vi "Preview Store.vi"(6 "Local Data in":T1, 7 "Action":enum16{"Open", "Get", "Close"}(ring)=enum."Get", 8 "error in (no error)":errorcluster, 10 "% resolution":i32=10) -> (2 "Image Store":T8[][](array[typedef]), 4 "Local Data out":T1)   [LabVIEW 2024]
uses:
  Controls/Test Cluster.ctl
  Controls/Excluded Information.ctl
  Controls/Language.ctl
  Controls/Device_Type.ctl
  <vilib>/Utility/miscctls.llb/LVRectTypeDef.ctl
  <vilib>/Utility/miscctls.llb/LVBoundsTypeDef.ctl
  Controls/RVHR - Local Data.ctl
  <vilib>/picture/picture.llb/imagedata.ctl
panel:
  out "2D Picture":picture
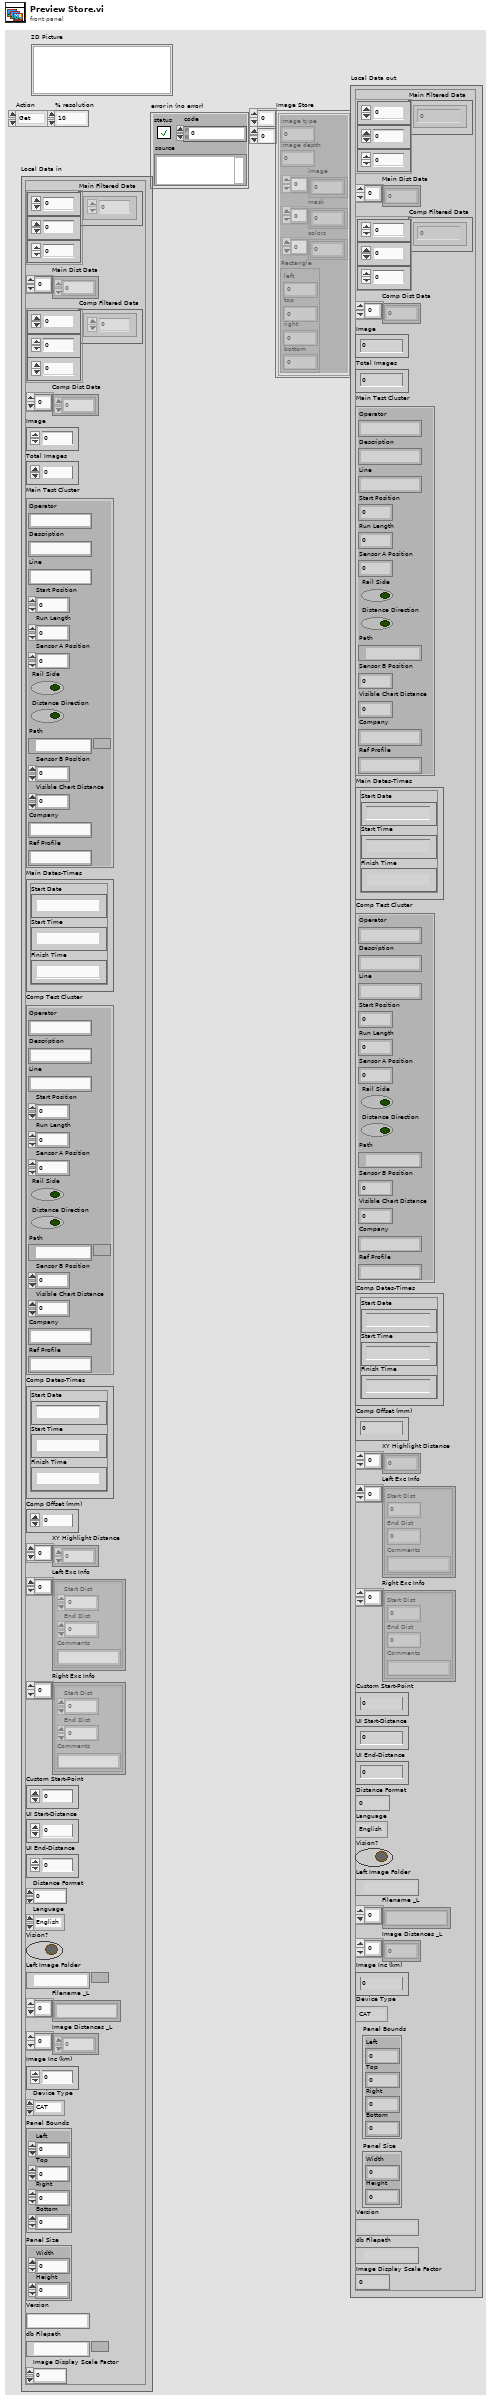
[diagram p1: front panel]
types:
  T1 = typedef "RVHR - Local Data.ctl" = cluster{"Main Filtered Data":dbl[][][], "Main Dist Data":dbl[], "Comp Filtered Data":dbl[][][], "Comp Dist Data":dbl[], "Image":u16, "Total Images":u16, "Main Test Cluster":T2, "Main Dates-Times":cluster{"Start Date":string, "Start Time":string, "Finish Time":string}, "Comp Test Cluster":T2, "Comp Dates-Times":cluster{"Start Date":string, "Start Time":string, "Finish Time":string}, "Comp Offset (mm)":i64, "XY Highlight Distance":dbl[], "Left Exc Info":T3[], "Right Exc Info":T3[], "Custom Start-Point":dbl, "UI Start-Distance":dbl, "UI End-Distance":dbl, "Distance Format":u8, "Language":T4, "Vision?":bool, "Left Image Folder":path, "Filename _L":string[], "Image Distances _L":dbl[], "Image Inc (km)":dbl, "Device Type":T5, "Panel Bounds":T6, "Panel Size":T7, "Version":string, "db Filepath":path, "Image Display Scale Factor":dbl}
  T2 = typedef "Test Cluster.ctl" = cluster{"Operator":string, "Description":string, "Line":string, "Start Position":dbl, "Run Length":dbl, "Sensor A Position":dbl, "Rail Side":bool, "Distance Direction":bool, "Path":path, "Sensor B Position":dbl, "Visible Chart Distance":dbl, "Company":string, "Ref Profile":string}
  T3 = typedef "Excluded Information.ctl" = cluster{"Start Dist":dbl, "End Dist":dbl, "Comments":string}
  T4 = typedef "Language.ctl" = enum16{"English", "Chinese", "German"}
  T5 = typedef "Device_Type.ctl" = enum16{"CAT", "Bi-CAT", "YRCA", "RCA", "RV-HR", "TV-HR"}
  T6 = typedef "LVRectTypeDef.ctl" = cluster{"Left":i16, "Top":i16, "Right":i16, "Bottom":i16}
  T7 = typedef "LVBoundsTypeDef.ctl" = cluster{"Width":u32, "Height":u32}
  T8 = typedef "imagedata.ctl" = cluster{"image type":i32, "image depth":i32, "image":u8[], "mask":u8[], "colors":u32[], "Rectangle":cluster{"left":i16, "top":i16, "right":i16, "bottom":i16}}
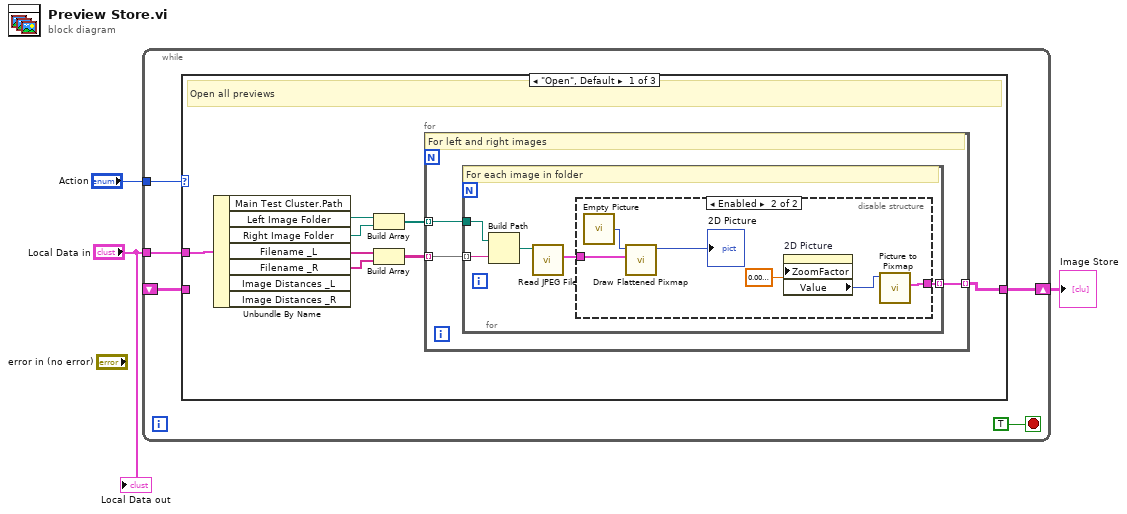
[diagram p0: block diagram]
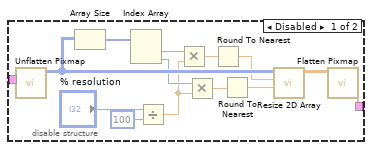
[diagram p2: hidden frame]
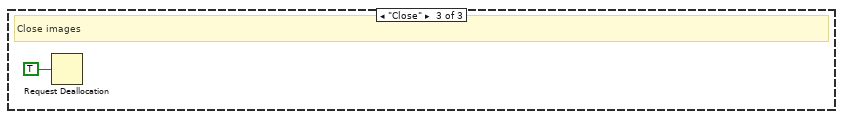
[diagram p4: hidden frame]
diagram:
  n1 = while {
    tunnel: "Action" -> [w8]
    tunnel: "Local Data in" -> [w7]
    shift-right: [w5] -> w1
    shift-left: _ -> [w4]
    stop <- TRUE stop-if-true
    n2 = case shown="\"Open\", Default" w8 {
      tunnel: w7 -> [w16 _ _]
      tunnel: [w9 w45 _] -> w5
      tunnel: w4 -> [_ w45 _]
      frame "Open", Default {
        # "Open all previews"
        n3 = Unbundle By Name(w16) -> ("Left Image Folder"=w12:path, "Right Image Folder"=w11:path, "Filename _L"=w15:string[], "Filename _R"=w14:string[])  [unwired: 3 out]
        n4 = Build Array(w12, w11) -> (w10:path[])
        n5 = Build Array(w15, w14) -> (w13:string[][])
        n6 = for {
          tunnel: w13 -> [w19] mode=indexing
          tunnel: w10 -> [w18] mode=indexing
          tunnel: [w17] -> w9 mode=indexing
          # "For left and right images"
          n7 = for {
            tunnel: w19 -> [w23] mode=indexing
            tunnel: w18 -> [w24]
            tunnel: [w20] -> w17 mode=indexing
            # "For each image in folder"
            n8 = Build Path(base path=w24, name or relative path=w23) -> (appended path=w22:path)
            n9 = call <vilib>:"Read JPEG File.vi"("path to JPEG file"=w22) -> ("image data"=w21:T8)  [unwired: 8 in, 2 out]
            n10 = disable-structure shown="Enabled" {
              disable-tunnel: w21 -> [w38 w44]
              disable-tunnel: [w36 w39] -> w20
              frame Disabled {
                n11 = call <vilib>:"Unflatten Pixmap.vi"("image data"=w38) -> ("24-bit pixmap"=w35:u32[][])  [unwired: 4 in, 6 out]
                n12 = Array Size(array=w35) -> (size(s)=w34:i32[])
                n13 = Index Array(array=w34) -> (element #1=w31:i32, element #2=w30:i32)  [unwired: 2 in]
                n14 = Divide(x="% resolution", y=100) -> (x/y=w29:dbl)
                n15 = Multiply(x=w31, y=w29) -> (x*y=w28:dbl)
                n16 = Multiply(x=w30, y=w29) -> (x*y=w27:dbl)
                n17 = Round To Nearest(number=w28) -> (nearest integer value=w25:dbl)
                n18 = Round To Nearest(number=w27) -> (nearest integer value=w26:dbl)
                n19 = call "Resize 2D Array.vi"("y dimension"=w26, "x dimension"=w25, "input array"=w35) -> ("output array"=w37:dbl[][])  [unwired: 8 in]
                n20 = call <vilib>:"Flatten Pixmap.vi"("24-bit pixmap"=w37) -> ("image data"=w36:T8)  [unwired: 10 in]
              }
              frame Enabled {
                n21 = call "Empty Picture"() -> ("empty picture"=w42:picture)
                n22 = call <vilib>:"Draw Flattened Pixmap.vi"("image data"=w44, "picture"=w42) -> ("new picture"=→"2D Picture":picture)  [unwired: 7 in]
                n23 = property on="2D Picture" class="Pict"("ZoomFactor"=sgl 0.01 ("Zoom Factor")) -> ("Value"=w40:picture)  [unwired: 2 in, 2 out]
                n24 = call <vilib>:"Picture to Pixmap.vi"("picture"=w40) -> ("image data"=w39:T8)  [unwired: 9 in, 1 out]
              }
            }
          }
        }
      }
      frame "Get" {
        # "Get current image preview"
      }
      frame "Close" {
        # "Close images"
        n25 = Request Deallocation(TRUE ("flag")) -> ()
      }
    }
  }
  "Image Store" <- w1
  "Local Data out" <- "Local Data in"
